vi "CSTK_BuildApplication_Manager_CreateZipFile.vi"(8 "错误输入（无错误）":errorcluster, 11 "BuildApplication Data in":T1={"Build Specification Name"="", "Destination Path"=path "", "Files Generated by Build"=[], "Exe Path Generated by Build"=path "", "Version"="", "Datatime"=timestamp(0 s since 1904-01-01), "ChangeLog"="", "Package as a ZIP file?"=TRUE, "Rename EXE File Name?"=FALSE, "Zip File Path"=path ""} {"Datatime" format="%<%.3X %x>T"}) -> (0 "错误输出":errorcluster, 3 "BuildApplication Data out":T1={"Build Specification Name"="", "Destination Path"=path "", "Files Generated by Build"=[], "Exe Path Generated by Build"=path "", "Version"="", "Datatime"=timestamp(0 s since 1904-01-01), "ChangeLog"="", "Package as a ZIP file?"=TRUE, "Rename EXE File Name?"=FALSE, "Zip File Path"=path ""} {"Datatime" format="%<%.3X %x>T"})   [LabVIEW 2015, in "CSTK_BuildApplication_Manager.lvlib"]
uses:
  CSTK_BuildApplication_Manager.lvlib
  CSTK_BuildApplication_Manager_data.ctl
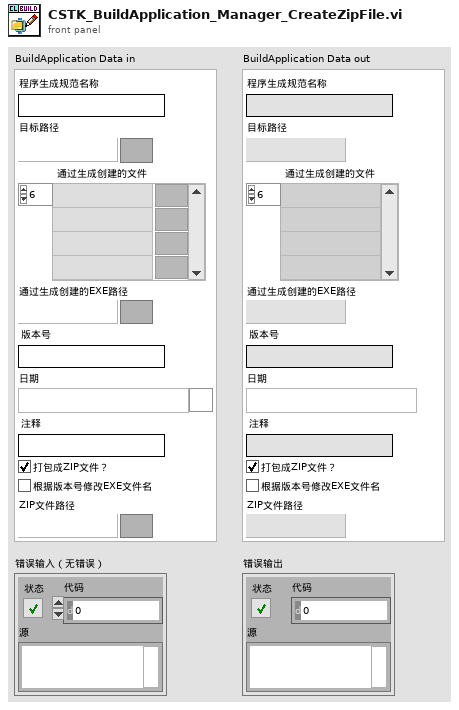
[diagram p1: front panel]
types:
  T1 = typedef "CSTK_BuildApplication_Manager.lvlib/CSTK_BuildApplication_Manager_data.ctl" = cluster{"Build Specification Name":string, "Destination Path":path, "Files Generated by Build":path[], "Exe Path Generated by Build":path, "Version":string, "Datatime":timestamp, "ChangeLog":string, "Package as a ZIP file?":bool, "Rename EXE File Name?":bool, "Zip File Path":path}
  T2 = enum16{"open", "replace", "create", "open or create", "replace or create", "replace or create with confirmation"}
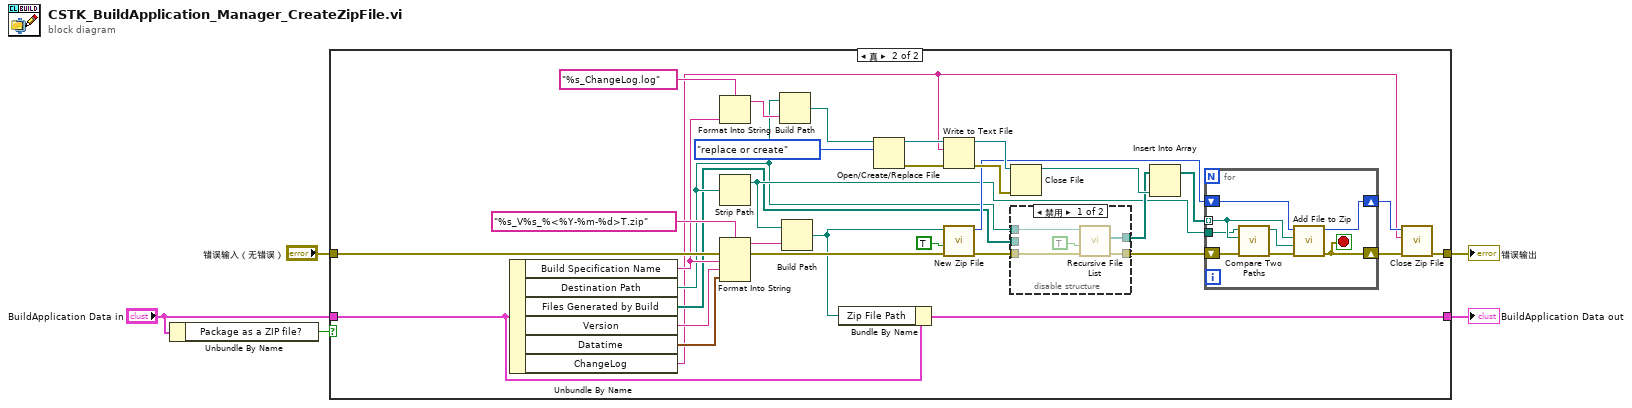
[diagram p0: block diagram]
diagram:
  n1 = Unbundle By Name("BuildApplication Data in") -> ("Package as a ZIP file?"=w1:bool)
  n2 = case shown="真" w1 {
    tunnel: "错误输入（无错误）" -> [w6 w28]
    tunnel: [w6 w27] -> w4
    tunnel: "BuildApplication Data in" -> [w7 w17]
    tunnel: [w7 w9] -> w3
    frame False {
    }
    frame True {
      n3 = Unbundle By Name(w17) -> ("Build Specification Name"=w16:string, "Destination Path"=w14:path, "Files Generated by Build"=w13:path[], "Version"=w12:string, "Datatime"=w11:timestamp, "ChangeLog"=w10:string)
      n4 = Format Into String(format string="%s_ChangeLog.log" ("格式字符串"), w16) -> (resulting string=w32:string)  [unwired: 2 in, 1 out]
      n5 = Strip Path(path=w14) -> (stripped path=w15:path)  [unwired: 1 out]
      n6 = Format Into String(format string="%s_V%s_%<%Y-%m-%d>T.zip" ("格式字符串"), error in=w28, w16, w12, w11) -> (resulting string=w19:string, error out=w29:errorcluster)  [unwired: 1 in]
      n7 = Build Path(base path=w14, name or relative path=w32) -> (appended path=w33:path)
      n8 = Build Path(base path=w15, name or relative path=w19) -> (appended path=w8:path)
      n9 = Bundle By Name(cluster=w17, "Zip File Path"=w8) -> (w9:T1)
      n10 = Open/Create/Replace File(file path (use dialog)=w33, operation (0:open)=T2."replace or create" ("操作(0:open)")) -> (refnum out=w36:refnum<file>, error out=w34:errorcluster)  [unwired: 4 in, 1 out]
      n11 = Write to Text File(file (use dialog)=w36, text=w10, error in=w34) -> (refnum out=w37:refnum<file>, error out=w35:errorcluster)  [unwired: 1 in, 1 out]
      n12 = call <vilib>:"New Zip File.vi"("error in (no error)"=w29, "confirm overwrite? (F)"=TRUE, "target"=w8) -> ("error out"=w22:errorcluster, "zip file out"=w20:i64)  [unwired: 2 in, 1 out]
      n13 = Close File(refnum=w37, error in=w35) -> (path=w39:path)  [unwired: 1 out]
      n14 = disable-structure shown="禁用" {
        disable-tunnel: w22 -> [w43 w46]
        disable-tunnel: [w42 w46] -> w23
        disable-tunnel: [w41 w45] -> w24
        disable-tunnel: w14 -> [w40 _]
        disable-tunnel: w13 -> [_ w45]
        frame Disabled {
          n15 = call <vilib>:"Recursive File List.vi"("error in (no error)"=w43, "Continue Recursing on Error? (F)"=TRUE, "Folder Path"=w40) -> ("error out"=w42:errorcluster, "All Files in Dir"=w41:path[])  [unwired: 4 in, 3 out]
        }
        frame Enabled {
        }
      }
      n16 = Insert Into Array(array=w24, new element=w39) -> (w38:path[])  [unwired: 1 in]
      n17 = for {
        shift-right: [w53] -> w25
        shift-left: w20 -> [w54]
        shift-right: [w47] -> w26
        shift-left: w23 -> [w50]
        tunnel: w38 -> [w52] mode=indexing
        tunnel: w15 -> [w51]
        stop <- w47 stop-if-true
        n18 = call <vilib>:"Compare Two Paths.vi"("error in (no error)"=w50, "Path 2"=w52, "Path 1"=w51) -> ("error out"=w49:errorcluster, "Relative Path from 1 to 2"=w48:path)  [unwired: 5 in, 2 out]
        n19 = call <vilib>:"Add File to Zip.vi"("error in (no error)"=w49, "destination path in zip"=w48, "source file path"=w52, "zip file in"=w54) -> ("error out"=w47:errorcluster, "zip file out"=w53:i64)  [unwired: 6 in]
      }
      n20 = call <vilib>:"Close Zip File.vi"("error in (no error)"=w26, "comments"=w10, "zip file in"=w25) -> ("error out"=w27:errorcluster)  [unwired: 4 out]
    }
  }
  "错误输出" <- w4
  "BuildApplication Data out" <- w3
